vi "GetPID.vi"(8 "error in (no error)":errorcluster, 11 "MotorCtrl in":refnum<class "MotorControl.lvclass">) -> (0 "error out":errorcluster, 2 "PID gain schedule":T1(array[cluster]), 3 "MotorCtrl out":refnum<class "MotorControl.lvclass">)   [LabVIEW 2015, in "MotorControl.lvclass"]
uses:
  MotorControl.lvclass
  MotorControl.lvclass/MotorControl.ctl
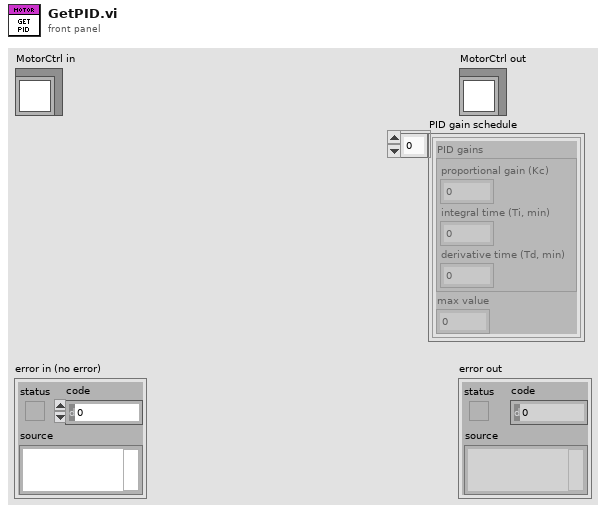
[diagram p1: front panel]
types:
  T1 = cluster{"PID gains":cluster{"proportional gain (Kc)":dbl, "integral time (Ti, min)":dbl, "derivative time (Td, min)":dbl}, "max value":dbl}[]
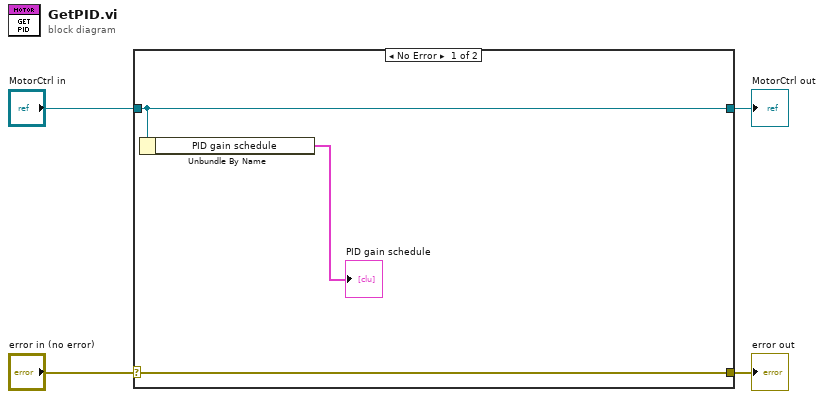
[diagram p0: block diagram]
diagram:
  n1 = case shown="No Error" "error in (no error)" {
    selector: "error in (no error)" -> [w7 w9]
    tunnel: [w7 w9] -> w3
    tunnel: [w6 w8] -> w1
    tunnel: "MotorCtrl in" -> [w6 w8]
    frame No Error {
      n2 = Unbundle By Name(w6) -> ("PID gain schedule"=→"PID gain schedule":T1)
    }
    frame Error {
    }
  }
  "error out" <- w3
  "MotorCtrl out" <- w1
